vi "Clear Pins SubVI.vi"(8 "Clear Pin Task In":refnum<k21>, 10 "Sync Pin Task In":refnum<k21>) -> (0 "Clear Pin Task Out":refnum<k21>, 2 "Sync Pin Task Out":refnum<k21>)   [LabVIEW 2020]
uses:
  <vilib>/DAQmx/write.llb/DAQmx Write (Digital Bool 1Line 1Point).vi
  <vilib>/DAQmx/miscellaneous.llb/DAQmx Fill In Error Info.vi
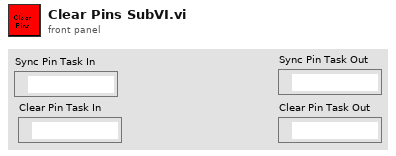
[diagram p1: front panel]
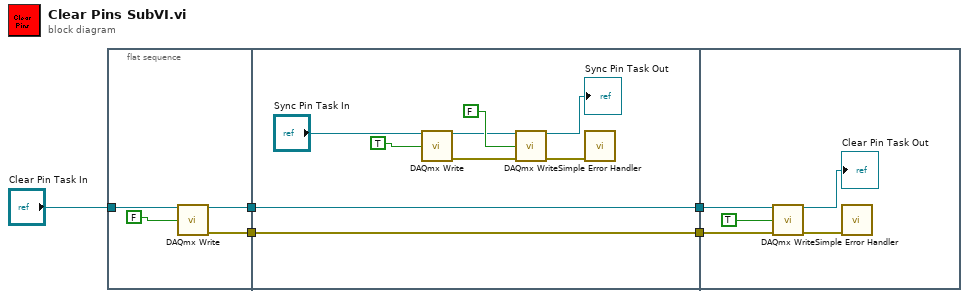
[diagram p0: block diagram]
diagram:
  n1 = flat-sequence {
    tunnel: "Clear Pin Task In" -> [w6]
    tunnel: [w8] -> w4
    tunnel: [w7] -> w2
    tunnel: w4 -> [w12]
    tunnel: [w12] -> w3
    tunnel: w2 -> [w11]
    tunnel: [w11] -> w1
    tunnel: w3 -> [w19]
    tunnel: w1 -> [w20]
    frame #0 {
      n2 = call-poly <vilib>:"DAQmx Write.vi"("task/channels in"=w6, "data"=FALSE) -> ("task out"=w7:refnum<k21>, "error out"=w8:errorcluster)  [unwired: 11 in, 1 out]
    }
    frame #1 {
      n3 = call-poly <vilib>:"DAQmx Write.vi"("task/channels in"="Sync Pin Task In", "data"=TRUE) -> ("task out"=w13:refnum<k21>, "error out"=w14:errorcluster)  [unwired: 11 in, 1 out]
      n4 = call-poly <vilib>:"DAQmx Write.vi"("task/channels in"=w13, "data"=FALSE, "error in"=w14) -> ("task out"=→"Sync Pin Task Out":refnum<k21>, "error out"=w15:errorcluster)  [unwired: 10 in, 1 out]
      n5 = call <vilib>:"Simple Error Handler.vi"("error in (no error)"=w15) -> ()  [unwired: 4 in, 5 out]
    }
    frame #2 {
      n6 = call-poly <vilib>:"DAQmx Write.vi"("task/channels in"=w20, "data"=TRUE, "error in"=w19) -> ("task out"=→"Clear Pin Task Out":refnum<k21>, "error out"=w21:errorcluster)  [unwired: 10 in, 1 out]
      n7 = call <vilib>:"Simple Error Handler.vi"("error in (no error)"=w21) -> ()  [unwired: 4 in, 5 out]
    }
  }
